vi "FetchImageSet (SubVI).vi"(8 "error in (no error)":errorcluster, 10 "Naming Convention":string="*.png", 11 "Images Directory":path=path "E:/XYZstage+Camera_CollectedImages/12-16-2016/noStaveMount/toolingpins_images") -> (0 "error out":errorcluster, 2 "Image Array":T1[](array[typedef]), 3 "Filenames Array":string[](array[string]))   [LabVIEW 2016]
uses:
  <vilib>/vision/Image Controls.llb/IMAQ Image.ctl
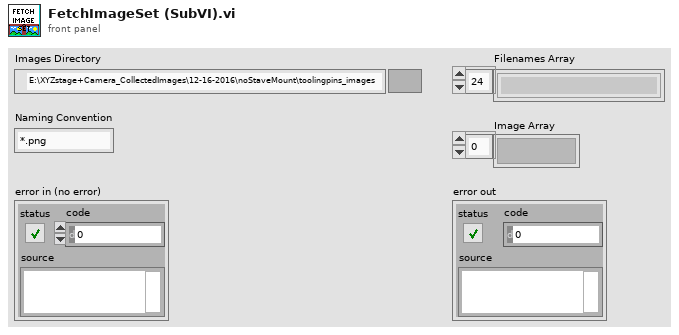
[diagram p1: front panel]
types:
  T1 = typedef "IMAQ Image.ctl" = refnum<image>
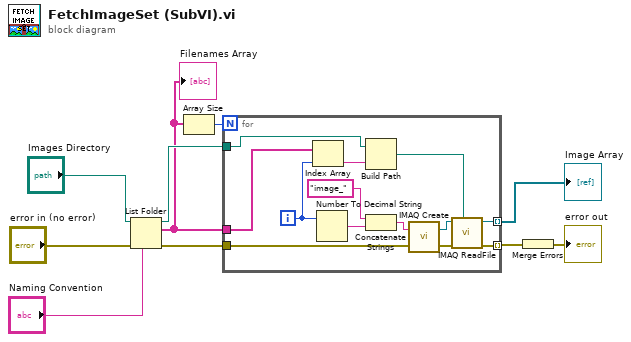
[diagram p0: block diagram]
diagram:
  n1 = List Folder(path="Images Directory", pattern="Naming Convention", error in="error in (no error)") -> (path out=w6:path, filenames=w5:string[], error out=w7:errorcluster)  [unwired: 1 in, 1 out]
  "Filenames Array" <- w5
  n2 = Array Size(array=w5) -> (size(s)=w4:i32)
  n3 = for {
    N: w4 -> [_]
    tunnel: w5 -> [w23]
    tunnel: w6 -> [w22]
    tunnel: w7 -> [w13]
    tunnel: [w12] -> w9 mode=indexing
    tunnel: [w11] -> w8 mode=indexing
    i -> [w20]
    n4 = Index Array(array=w23, index=w20) -> (element=w21:string)
    n5 = Number To Decimal String(number=w20) -> (decimal integer string=w19:string)  [unwired: 1 in]
    n6 = Build Path(base path=w22, name or relative path=w21) -> (appended path=w15:path)
    n7 = Concatenate Strings("image_" ("string"), w19) -> (w14:string)
    n8 = call "IMAQ Create"("Image Name"=w14, "error in (no error)"=w13) -> ("New Image"=w16:T1, "error out"=w17:errorcluster)  [unwired: 3 in]
    n9 = call "IMAQ ReadFile"("File Path"=w15, "error in (no error)"=w17, "Image"=w16) -> ("error out"=w11:errorcluster, "Image Out"=w12:T1)  [unwired: 4 in, 3 out]
  }
  "Image Array" <- w9
  n10 = Merge Errors(w8) -> (→"error out":errorcluster)
